vi "Pitch data.vi"(0 "Test Graph":refnum<vi>[](array[refnum]), 1 "Tab_Graph":refnum<vi>, 2 "Frequency(Hz)":dbl[](array[numeric]), 3 "Diff S-parameters  Data":dbl[][](array[numeric]), 5 "Selected Test Item":string[](array[string])=["SDD21", "SDD22", "SCD21", "SCD22", "SCC11", "SCC22"], 9 "Spec Association Col No":string[](array[string])=["1", "2", "3", "4", "NAN", "NAN", "NAN", "NAN"], 11 "Spec _Data":dbl[][](array[numeric])) -> (20 "Data out":T1(array[cluster]))   [LabVIEW 2011]
panel:
  in  "All Diff  Test  Item":string[](array[string])=["SDD21", "SDD12", "SDD11", "SDD22", "SCD21", "SCD12", "SCD22", "SCD11", "SDC11", "SDC22", "SDC12", "SDC21", "SCC11", "SCC22", "SCC12", "SCC21"]
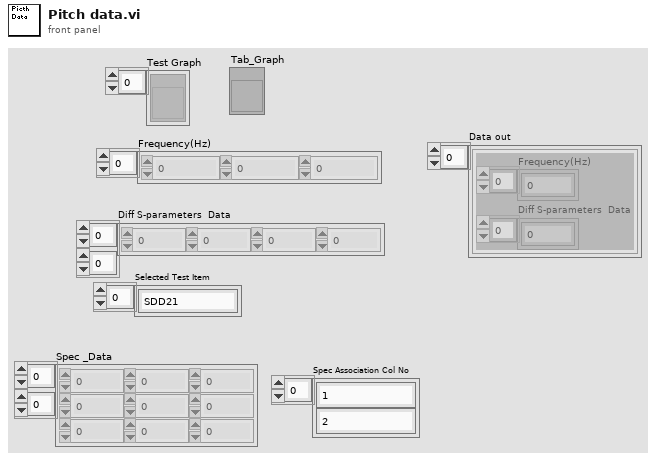
[diagram p1: front panel]
types:
  T1 = cluster{"Frequency(Hz)":dbl[], "Diff S-parameters  Data":dbl[]}[]
  T2 = cluster{"Frequency(Hz)":dbl[], "Diff S-parameters  Data":dbl[]}
  T3 = cluster{"Frequency(Hz)":dbl[], "Spec _Data":dbl[]}
  T4 = cluster{"Frequency(Hz)":dbl[], "Spec _Data":dbl[]}[]
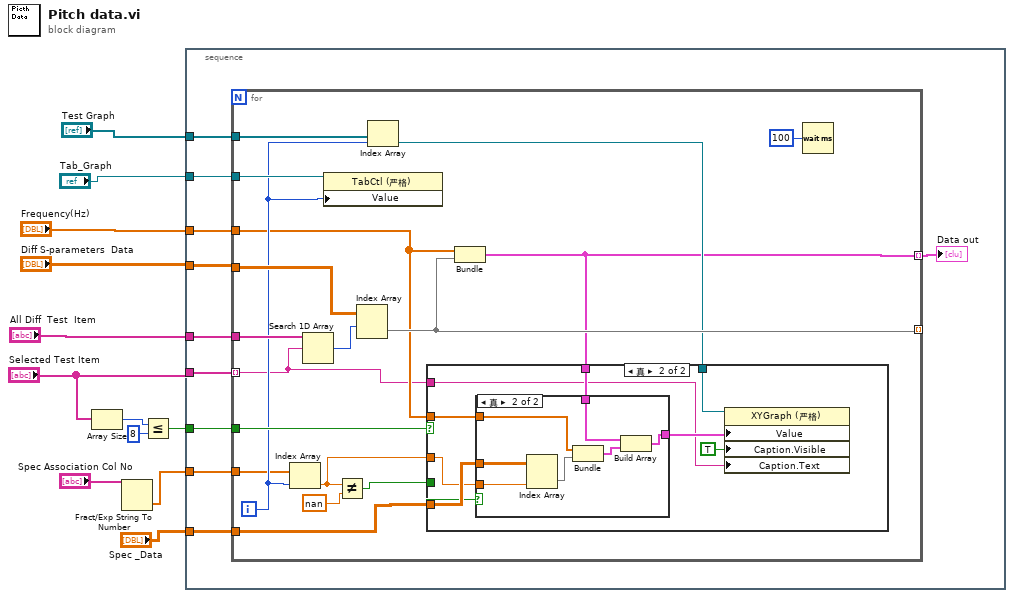
[diagram p0: block diagram]
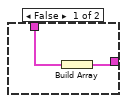
[diagram p3: hidden frame]
diagram:
  n1 = Array Size(array="Selected Test Item") -> (size(s)=w7:i32)
  n2 = Fract/Exp String To Number(string="Spec Association Col No") -> (number=w3:dbl[])  [unwired: 3 in, 1 out]
  n3 = Less Or Equal?(x=w7, y=8) -> (x <= y?=w5:bool)
  n4 = stacked-sequence {
    tunnel: "All Diff  Test  Item" -> [w22]
    tunnel: "Diff S-parameters  Data" -> [w21]
    tunnel: "Selected Test Item" -> [w20]
    tunnel: "Frequency(Hz)" -> [w19]
    tunnel: "Test Graph" -> [w18]
    tunnel: "Tab_Graph" -> [w16]
    tunnel: w5 -> [w15]
    tunnel: w3 -> [w14]
    tunnel: "Spec _Data" -> [w13]
    frame #0 {
      n5 = for {
        tunnel: w20 -> [w23] mode=indexing
        tunnel: w22 -> [w40]
        tunnel: w21 -> [w39]
        tunnel: [w36] -> _ mode=indexing
        tunnel: w18 -> [w37]
        tunnel: w19 -> [w24]
        tunnel: [w34] -> w17 mode=indexing
        tunnel: w16 -> [w33]
        tunnel: w15 -> [w31]
        tunnel: w14 -> [w29]
        tunnel: w13 -> [w26]
        i -> [w30]
        n6 = Index Array(array=w29, index=w30) -> (element=w25:dbl)
        n7 = Search 1D Array(1D array=w40, element=w23) -> (index of element=w38:i32)  [unwired: 1 in]
        n8 = property class="TabCtl (严格)"(reference=w33, "Value"=w30) -> ()  [unwired: 1 in, 2 out]
        n9 = Not Equal?(x=w25, y=nan) -> (x != y?=w27:bool)
        n10 = Index Array(array=w39, index (row)=w38) -> (element=w36:dbl[])  [unwired: 1 in]
        n11 = Index Array(array=w37, index=w30) -> (element=w35:refnum<vi>)
        n12 = Bundle("Frequency(Hz)"=w24, "Diff S-parameters  Data"=w36) -> (w34:T2)  [unwired: 1 in]
        n13 = case shown="真" w31 {
          tunnel: w35 -> [_ w49]
          tunnel: w34 -> [_ w44]
          tunnel: w27 -> [_ w46]
          tunnel: w26 -> [_ w48]
          tunnel: w25 -> [_ w47]
          tunnel: w24 -> [_ w45]
          tunnel: w23 -> [_ w41]
          frame False {
          }
          frame True {
            n14 = case shown="真" w46 {
              tunnel: w48 -> [_ w58]
              tunnel: w47 -> [_ w57]
              tunnel: w45 -> [_ w55]
              tunnel: w44 -> [w51 w53]
              tunnel: [w50 w52] -> w43
              frame False {
                n15 = Build Array(w51) -> (w50:T1)
              }
              frame True {
                n16 = Index Array(array=w58, index (col)=w57) -> (element=w56:dbl[])  [unwired: 1 in]
                n17 = Bundle("Frequency(Hz)"=w55, "Spec _Data"=w56) -> (w54:T3)  [unwired: 1 in]
                n18 = Build Array(w53, w54) -> (w52:T4)
              }
            }
            n19 = property class="XYGraph (严格)"(reference=w49, "Value"=w43, "Caption.Visible"=TRUE ("标题.可见"), "Caption.Text"=w41) -> ()  [unwired: 1 in, 2 out]
          }
        }
        n20 = Wait (ms)(milliseconds to wait=u32 100 ("等待时间（毫秒）")) -> ()  [unwired: 1 out]
      }
      "Data out" <- w17
    }
  }
